vi "6229_Green_Lattice_write_waveform_2015.10.19.vi"(8 "Error In":errorcluster, 9 "Control Reference \nCluster Input":T1, 11 "6229 Green Lattice Inputs":T2={"Active Device"="6229_Green_Lattice", "Active Channels"=[TRUE, TRUE, TRUE, TRUE, FALSE, FALSE, FALSE, FALSE], "Active Phases"=[TRUE, FALSE, FALSE, FALSE, FALSE, FALSE], "Phase Times"=[1.0, 0.1, 0.1], "Trigger Channel"="/6229_Green_Lattice/PFI0", "FIFO Buffer Size"=8191.0, "Sample Step Time (us)"=0.0, "Initialization Parameters"={"Enable Initialization"=FALSE, "Initial Values"=[]}, "Waveform Parameters"=[[{"Initial Value"=1.0, "Final Value"=0.0, "Tau"=0.0, "Eta"=1.0, "Nickname"="", "Function Type"=enum."Power Law", "Conversion"=enum."B Field Grad (G/cm)", "Constant"=0.0}, {"Initial Value"=1.0, "Final Value"=0.0, "Tau"=0.0, "Eta"=1.0, "Nickname"="", "Function Type"=enum."Power Law", "Conversion"=enum."B Field Grad (G/cm)", "Constant"=0.0}, {"Initial Value"=1.0, "Final Value"=0.0, "Tau"=0.0, "Eta"=1.0, "Nickname"="", "Function Type"=enum."Power Law", "Conversion"=enum."B Field Grad (G/cm)", "Constant"=0.0}, {"Initial Value"=1.0, "Final Value"=0.0, "Tau"=0.0, "Eta"=1.0, "Nickname"="", "Function Type"=enum."Power Law", "Conversion"=enum."B Field Grad (G/cm)", "Constant"=0.0}, {"Initial Value"=1.0, "Final Value"=0.0, "Tau"=0.0, "Eta"=1.0, "Nickname"="", "Function Type"=enum."Power Law", "Conversion"=enum."B Field Grad (G/cm)", "Constant"=0.0}, {"Initial Value"=1.0, "Final Value"=0.0, "Tau"=0.0, "Eta"=1.0, "Nickname"="", "Function Type"=enum."Power Law", "Conversion"=enum."B Field Grad (G/cm)", "Constant"=0.0}], [{"Initial Value"=1.0, "Final Value"=0.0, "Tau"=0.0, "Eta"=1.0, "Nickname"="", "Function Type"=enum."Power Law", "Conversion"=enum."B Field Grad (G/cm)", "Constant"=0.0}, {"Initial Value"=1.0, "Final Value"=0.0, "Tau"=0.0, "Eta"=1.0, "Nickname"="", "Function Type"=enum."Power Law", "Conversion"=enum."B Field Grad (G/cm)", "Constant"=0.0}, {"Initial Value"=1.0, "Final Value"=0.0, "Tau"=0.0, "Eta"=1.0, "Nickname"="", "Function Type"=enum."Power Law", "Conversion"=enum."B Field Grad (G/cm)", "Constant"=0.0}, {"Initial Value"=1.0, "Final Value"=0.0, "Tau"=0.0, "Eta"=1.0, "Nickname"="", "Function Type"=enum."Power Law", "Conversion"=enum."B Field Grad (G/cm)", "Constant"=0.0}, {"Initial Value"=1.0, "Final Value"=0.0, "Tau"=0.0, "Eta"=1.0, "Nickname"="", "Function Type"=enum."Power Law", "Conversion"=enum."B Field Grad (G/cm)", "Constant"=0.0}, {"Initial Value"=1.0, "Final Value"=0.0, "Tau"=0.0, "Eta"=1.0, "Nickname"="", "Function Type"=enum."Power Law", "Conversion"=enum."B Field Grad (G/cm)", "Constant"=0.0}], [{"Initial Value"=1.0, "Final Value"=0.0, "Tau"=0.0, "Eta"=1.0, "Nickname"="", "Function Type"=enum."Power Law", "Conversion"=enum."B Field Grad (G/cm)", "Constant"=0.0}, {"Initial Value"=1.0, "Final Value"=0.0, "Tau"=0.0, "Eta"=1.0, "Nickname"="", "Function Type"=enum."Power Law", "Conversion"=enum."B Field Grad (G/cm)", "Constant"=0.0}, {"Initial Value"=1.0, "Final Value"=0.0, "Tau"=0.0, "Eta"=1.0, "Nickname"="", "Function Type"=enum."Power Law", "Conversion"=enum."B Field Grad (G/cm)", "Constant"=0.0}, {"Initial Value"=1.0, "Final Value"=0.0, "Tau"=0.0, "Eta"=1.0, "Nickname"="", "Function Type"=enum."Power Law", "Conversion"=enum."B Field Grad (G/cm)", "Constant"=0.0}, {"Initial Value"=1.0, "Final Value"=0.0, "Tau"=0.0, "Eta"=1.0, "Nickname"="", "Function Type"=enum."Power Law", "Conversion"=enum."B Field Grad (G/cm)", "Constant"=0.0}, {"Initial Value"=1.0, "Final Value"=0.0, "Tau"=0.0, "Eta"=1.0, "Nickname"="", "Function Type"=enum."Power Law", "Conversion"=enum."B Field Grad (G/cm)", "Constant"=0.0}], [{"Initial Value"=1.0, "Final Value"=0.0, "Tau"=0.0, "Eta"=1.0, "Nickname"="", "Function Type"=enum."Power Law", "Conversion"=enum."B Field Grad (G/cm)", "Constant"=0.0}, {"Initial Value"=1.0, "Final Value"=0.0, "Tau"=0.0, "Eta"=1.0, "Nickname"="", "Function Type"=enum."Power Law", "Conversion"=enum."B Field Grad (G/cm)", "Constant"=0.0}, {"Initial Value"=1.0, "Final Value"=0.0, "Tau"=0.0, "Eta"=1.0, "Nickname"="", "Function Type"=enum."Power Law", "Conversion"=enum."B Field Grad (G/cm)", "Constant"=0.0}, {"Initial Value"=1.0, "Final Value"=0.0, "Tau"=0.0, "Eta"=1.0, "Nickname"="", "Function Type"=enum."Power Law", "Conversion"=enum."B Field Grad (G/cm)", "Constant"=0.0}, {"Initial Value"=1.0, "Final Value"=0.0, "Tau"=0.0, "Eta"=1.0, "Nickname"="", "Function Type"=enum."Power Law", "Conversion"=enum."B Field Grad (G/cm)", "Constant"=0.0}, {"Initial Value"=1.0, "Final Value"=0.0, "Tau"=0.0, "Eta"=1.0, "Nickname"="", "Function Type"=enum."Power Law", "Conversion"=enum."B Field Grad (G/cm)", "Constant"=0.0}], [{"Initial Value"=1.0, "Final Value"=0.0, "Tau"=0.0, "Eta"=1.0, "Nickname"="", "Function Type"=enum."Power Law", "Conversion"=enum."B Field Grad (G/cm)", "Constant"=0.0}, {"Initial Value"=1.0, "Final Value"=0.0, "Tau"=0.0, "Eta"=1.0, "Nickname"="", "Function Type"=enum."Power Law", "Conversion"=enum."B Field Grad (G/cm)", "Constant"=0.0}, {"Initial Value"=1.0, "Final Value"=0.0, "Tau"=0.0, "Eta"=1.0, "Nickname"="", "Function Type"=enum."Power Law", "Conversion"=enum."B Field Grad (G/cm)", "Constant"=0.0}, {"Initial Value"=1.0, "Final Value"=0.0, "Tau"=0.0, "Eta"=1.0, "Nickname"="", "Function Type"=enum."Power Law", "Conversion"=enum."B Field Grad (G/cm)", "Constant"=0.0}, {"Initial Value"=1.0, "Final Value"=0.0, "Tau"=0.0, "Eta"=1.0, "Nickname"="", "Function Type"=enum."Power Law", "Conversion"=enum."B Field Grad (G/cm)", "Constant"=0.0}, {"Initial Value"=1.0, "Final Value"=0.0, "Tau"=0.0, "Eta"=1.0, "Nickname"="", "Function Type"=enum."Power Law", "Conversion"=enum."B Field Grad (G/cm)", "Constant"=0.0}], [{"Initial Value"=1.0, "Final Value"=0.0, "Tau"=0.0, "Eta"=1.0, "Nickname"="", "Function Type"=enum."Power Law", "Conversion"=enum."B Field Grad (G/cm)", "Constant"=0.0}, {"Initial Value"=1.0, "Final Value"=0.0, "Tau"=0.0, "Eta"=1.0, "Nickname"="", "Function Type"=enum."Power Law", "Conversion"=enum."B Field Grad (G/cm)", "Constant"=0.0}, {"Initial Value"=1.0, "Final Value"=0.0, "Tau"=0.0, "Eta"=1.0, "Nickname"="", "Function Type"=enum."Power Law", "Conversion"=enum."B Field Grad (G/cm)", "Constant"=0.0}, {"Initial Value"=1.0, "Final Value"=0.0, "Tau"=0.0, "Eta"=1.0, "Nickname"="", "Function Type"=enum."Power Law", "Conversion"=enum."B Field Grad (G/cm)", "Constant"=0.0}, {"Initial Value"=1.0, "Final Value"=0.0, "Tau"=0.0, "Eta"=1.0, "Nickname"="", "Function Type"=enum."Power Law", "Conversion"=enum."B Field Grad (G/cm)", "Constant"=0.0}, {"Initial Value"=1.0, "Final Value"=0.0, "Tau"=0.0, "Eta"=1.0, "Nickname"="", "Function Type"=enum."Power Law", "Conversion"=enum."B Field Grad (G/cm)", "Constant"=0.0}], [{"Initial Value"=1.0, "Final Value"=0.0, "Tau"=0.0, "Eta"=1.0, "Nickname"="", "Function Type"=enum."Power Law", "Conversion"=enum."B Field Grad (G/cm)", "Constant"=0.0}, {"Initial Value"=1.0, "Final Value"=0.0, "Tau"=0.0, "Eta"=1.0, "Nickname"="", "Function Type"=enum."Power Law", "Conversion"=enum."B Field Grad (G/cm)", "Constant"=0.0}, {"Initial Value"=1.0, "Final Value"=0.0, "Tau"=0.0, "Eta"=1.0, "Nickname"="", "Function Type"=enum."Power Law", "Conversion"=enum."B Field Grad (G/cm)", "Constant"=0.0}, {"Initial Value"=1.0, "Final Value"=0.0, "Tau"=0.0, "Eta"=1.0, "Nickname"="", "Function Type"=enum."Power Law", "Conversion"=enum."B Field Grad (G/cm)", "Constant"=0.0}, {"Initial Value"=1.0, "Final Value"=0.0, "Tau"=0.0, "Eta"=1.0, "Nickname"="", "Function Type"=enum."Power Law", "Conversion"=enum."B Field Grad (G/cm)", "Constant"=0.0}, {"Initial Value"=1.0, "Final Value"=0.0, "Tau"=0.0, "Eta"=1.0, "Nickname"="", "Function Type"=enum."Power Law", "Conversion"=enum."B Field Grad (G/cm)", "Constant"=0.0}], [{"Initial Value"=1.0, "Final Value"=0.0, "Tau"=0.0, "Eta"=1.0, "Nickname"="", "Function Type"=enum."Power Law", "Conversion"=enum."B Field Grad (G/cm)", "Constant"=0.0}, {"Initial Value"=1.0, "Final Value"=0.0, "Tau"=0.0, "Eta"=1.0, "Nickname"="", "Function Type"=enum."Power Law", "Conversion"=enum."B Field Grad (G/cm)", "Constant"=0.0}, {"Initial Value"=1.0, "Final Value"=0.0, "Tau"=0.0, "Eta"=1.0, "Nickname"="", "Function Type"=enum."Power Law", "Conversion"=enum."B Field Grad (G/cm)", "Constant"=0.0}, {"Initial Value"=1.0, "Final Value"=0.0, "Tau"=0.0, "Eta"=1.0, "Nickname"="", "Function Type"=enum."Power Law", "Conversion"=enum."B Field Grad (G/cm)", "Constant"=0.0}, {"Initial Value"=1.0, "Final Value"=0.0, "Tau"=0.0, "Eta"=1.0, "Nickname"="", "Function Type"=enum."Power Law", "Conversion"=enum."B Field Grad (G/cm)", "Constant"=0.0}, {"Initial Value"=1.0, "Final Value"=0.0, "Tau"=0.0, "Eta"=1.0, "Nickname"="", "Function Type"=enum."Power Law", "Conversion"=enum."B Field Grad (G/cm)", "Constant"=0.0}]]} {"Phase Times" format="%_3p"}) -> (0 "error out":errorcluster, 2 "counter task out":refnum<k21>, 3 "waveform task out":refnum<k21>)   [LabVIEW 2016]
uses:
  Controls/6229/6229_arb_waveform_generation.ctl
  Controls/6229/6229_evap_waveform_input.ctl
  6221 arb waveforms/6221_waveform_param.ctl
  6733_Red_MOT/Neutral_voltage_conversion_control.ctl
  6733 arb waveforms/Control 1.ctl
  <vilib>/DAQmx/write.llb/DAQmx Write (Analog 1D DBL NChan 1Samp).vi
  <vilib>/DAQmx/write.llb/DAQmx Write (Analog 1D Wfm NChan NSamp).vi
  <vilib>/DAQmx/create/channels.llb/DAQmx Create Channel (AO-Voltage-Basic).vi
  <vilib>/DAQmx/miscellaneous.llb/DAQmx Fill In Error Info.vi
  <vilib>/Waveform/WDTOps.llb/WDT Append Waveforms DBL.vi
  <vilib>/Waveform/WDTOps.llb/WDT Scale Delta t DBL.vi
  <vilib>/DAQmx/configure/timing.llb/DAQmx Timing (Sample Clock).vi
  <vilib>/DAQmx/create/channels.llb/DAQmx Create Channel (CO-Pulse Generation-Frequency).vi
  <vilib>/DAQmx/configure/timing.llb/DAQmx Timing (Implicit).vi
  <vilib>/DAQmx/configure/trigger.llb/DAQmx Start Trigger (Digital Edge).vi
  <resource>/objmgr/daqmx.rc
panel:
  out "Sample Time Delta (us)":dbl
  out "Total Time":dbl
  out "Sample Rate":dbl
  out "Waveforms":waveform(dbl)[](array[waveform])
  out "Max Sample Rate":dbl=1000000.0
  out "# Inactive Channels":i32
  out "# Active Channels":i16
  out "Inactive Channels":tag[](array[tag])
  out "Active Channels":tag[](array[tag])
  out "Samples Written":dbl
  out "Voltage Maximum":dbl
  out "Voltage Minimum":dbl
  out "AO.PhysicalChans":tag[](array[tag])
  out "Active Device":tag
  # "(0) Arm A"
  # "(1) Arm B"
  # "(2) Arm C"
  # "(3) Unused"
  # "(0) Arm A"
  # "(1) Arm B"
  # "(2) Arm C"
  # "(3) Unused"
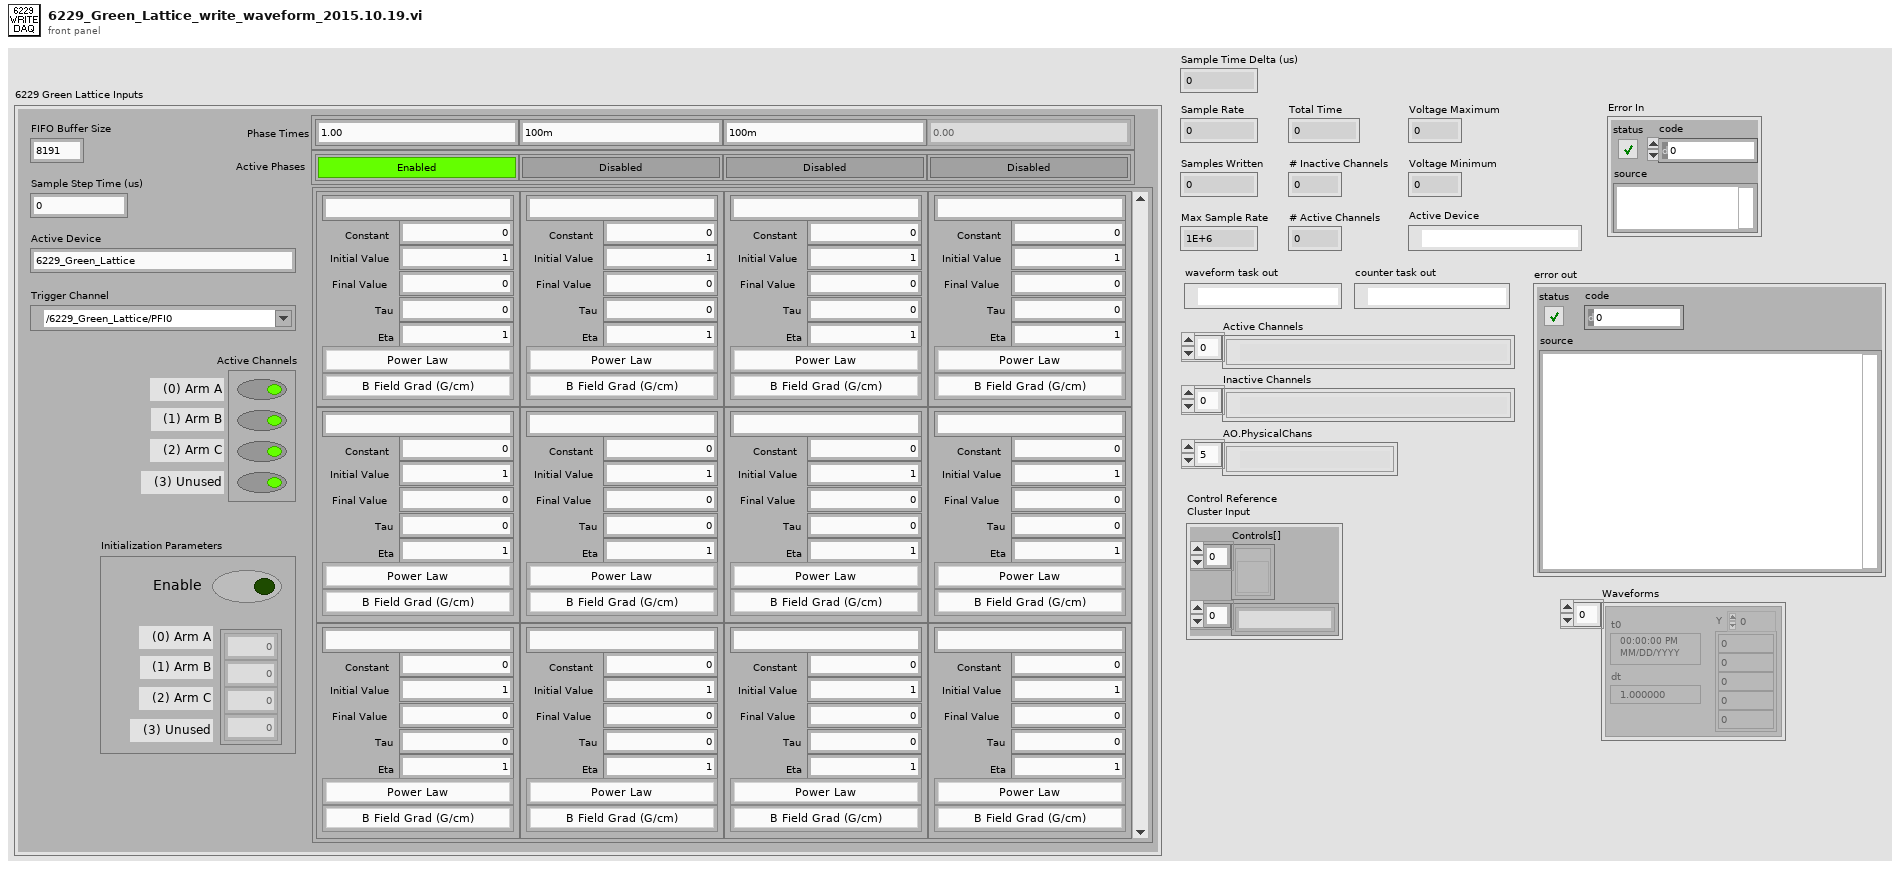
[diagram p1: front panel]
types:
  T1 = cluster{"Controls[]":refnum<vi>[], "Control Names":string[]}
  T2 = typedef "6229_arb_waveform_generation.ctl" = cluster{"Active Device":string, "Active Channels":bool[], "Active Phases":bool[], "Phase Times":dbl[], "Trigger Channel":tag, "FIFO Buffer Size":dbl, "Sample Step Time (us)":dbl, "Initialization Parameters":cluster{"Enable Initialization":bool, "Initial Values":dbl[]}, "Waveform Parameters":T3}
  T3 = typedef "6229_evap_waveform_input.ctl" = T4[][]
  T4 = typedef "6221_waveform_param.ctl" = cluster{"Initial Value":dbl, "Final Value":dbl, "Tau":dbl, "Eta":dbl, "Nickname":string, "Function Type":enum16{"Constant", "Power Law", "Evap - Calc Tau", "Evaporation Formula", "Tanh", "Exponential"}, "Conversion":T5, "Constant":dbl}
  T5 = typedef "Neutral_voltage_conversion_control.ctl" = enum16{"Volts", "B Field Grad (G/cm)", "Red Boson Cntr Freq (MHz)", "Red Boson Dither Amp (kHz)", "Red Boson Power (mW)", "Red 87 Trap Cntr Freq (MHz)", "Red 87 Trap Dither Amp (kHz)", "Red 87 Trap Power (mW)", "Red 87 Stir Cntr Freq (MHz)", "Red 87 Stir Dither Amp (kHz)", "Red 87 Stir Power (mW)", "ODT Sheet Trap Power (W)", "ODT Loading Trap Power (W)"}
  T6 = typedef "Control 1.ctl" = enum16{"Initialize", "Get Device Information", "Get Active/Inactive Channels", "Maximize Samples / Channel", "Calculate Waveforms", "Check for Problems", "Update Front Panel", "Clear Old Tasks", "Write Initialization to Cards", "Write Waveform to Cards"}
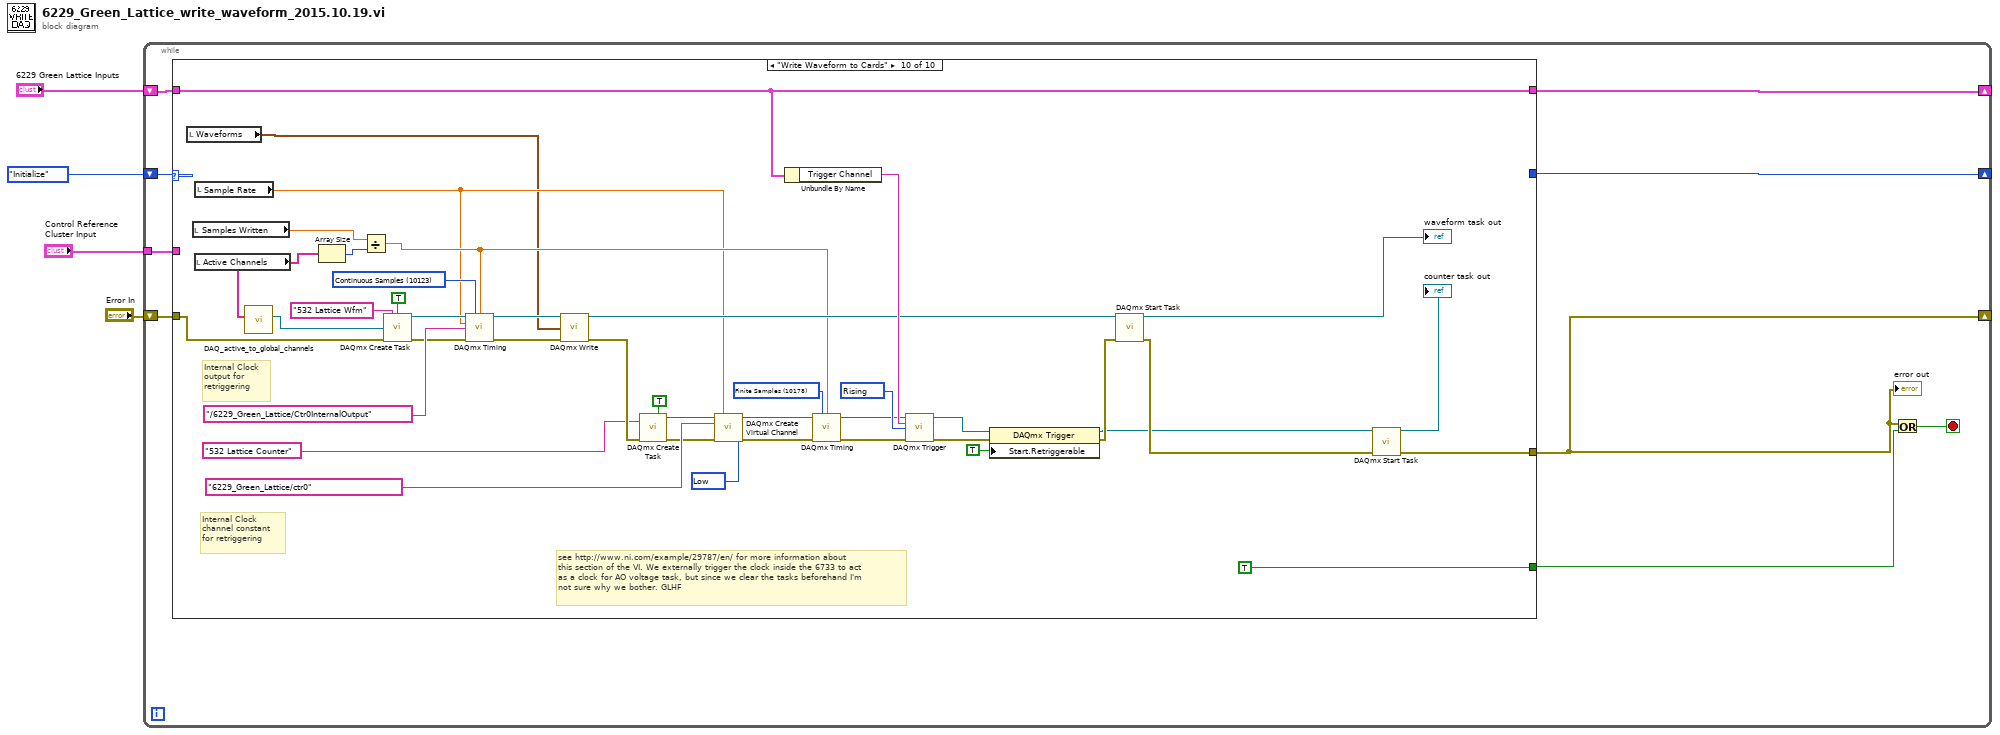
[diagram p0: block diagram]
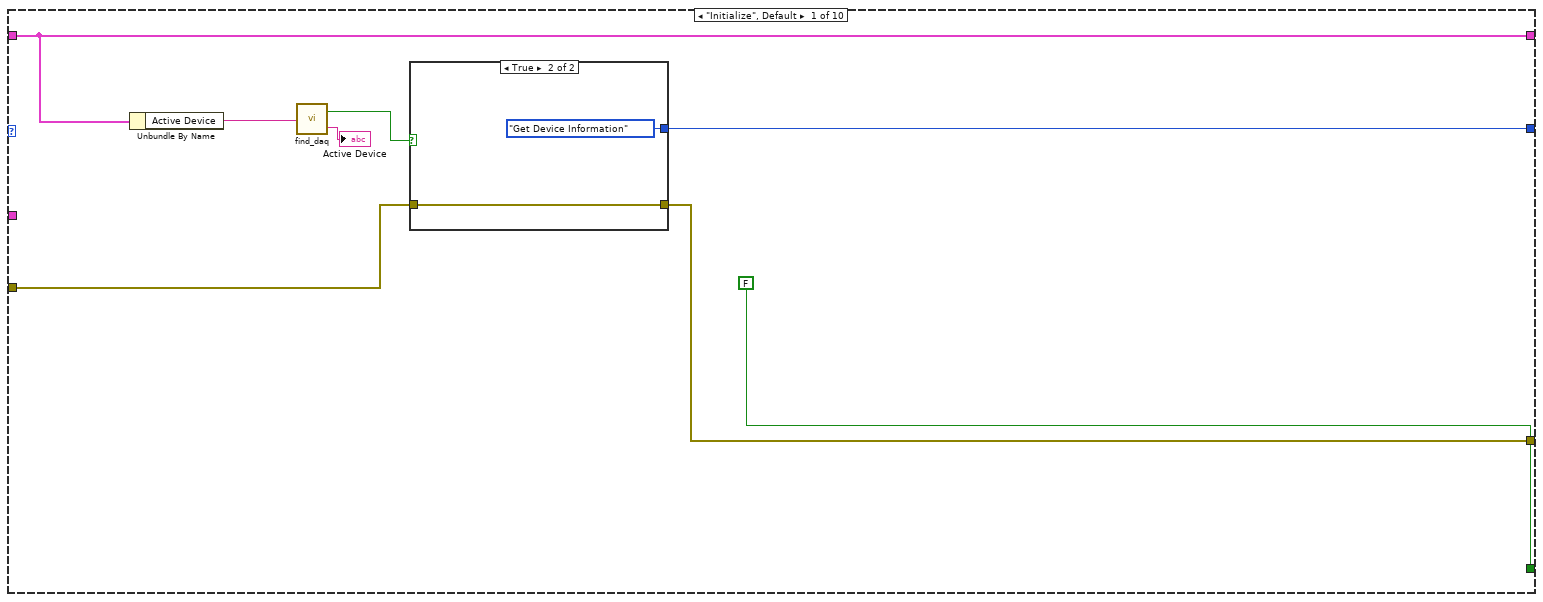
[diagram p2: hidden frame]
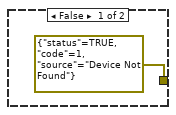
[diagram p3: hidden frame]
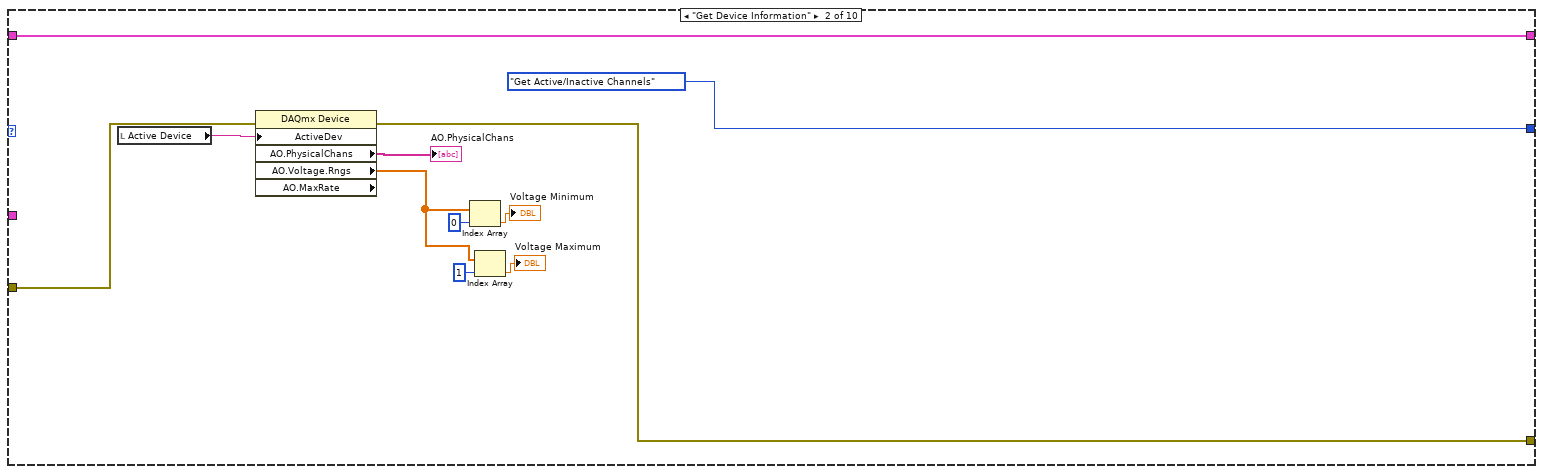
[diagram p4: hidden frame]
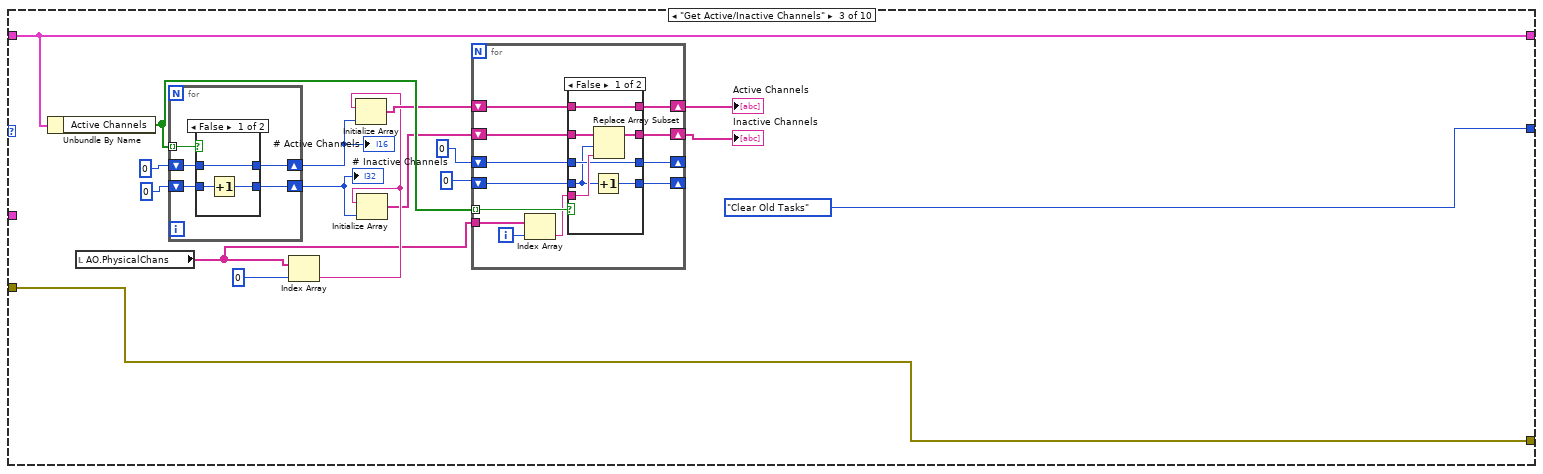
[diagram p5: hidden frame]
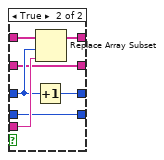
[diagram p6: hidden frame]
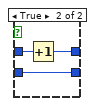
[diagram p7: hidden frame]
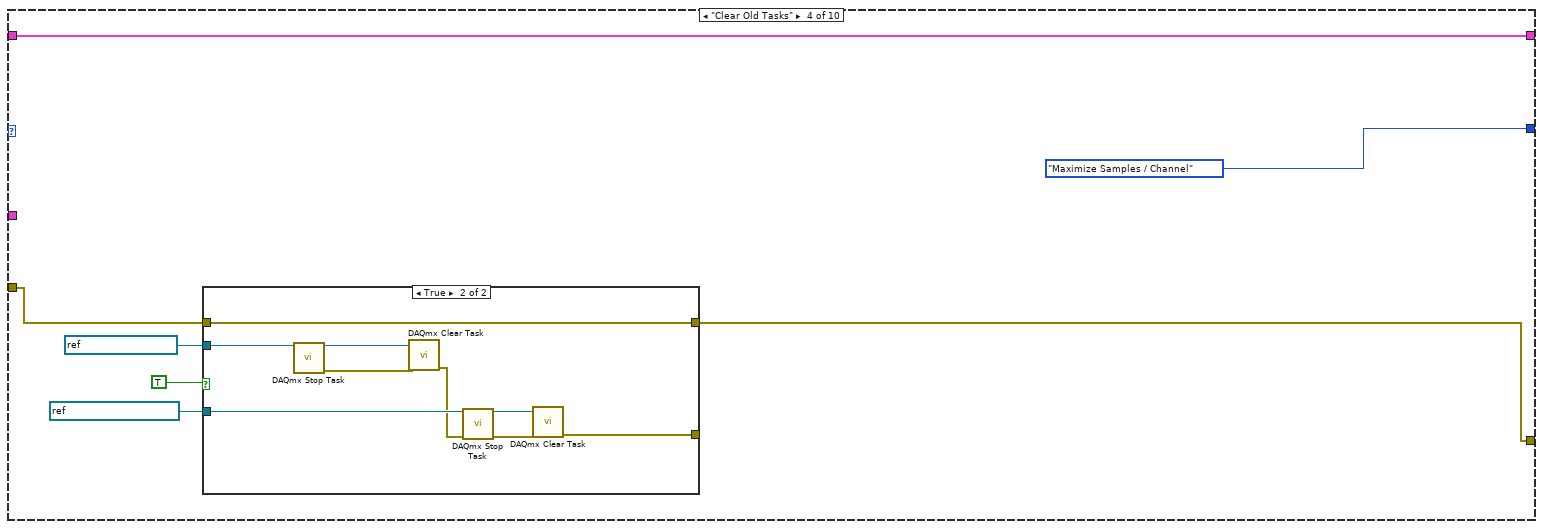
[diagram p8: hidden frame]
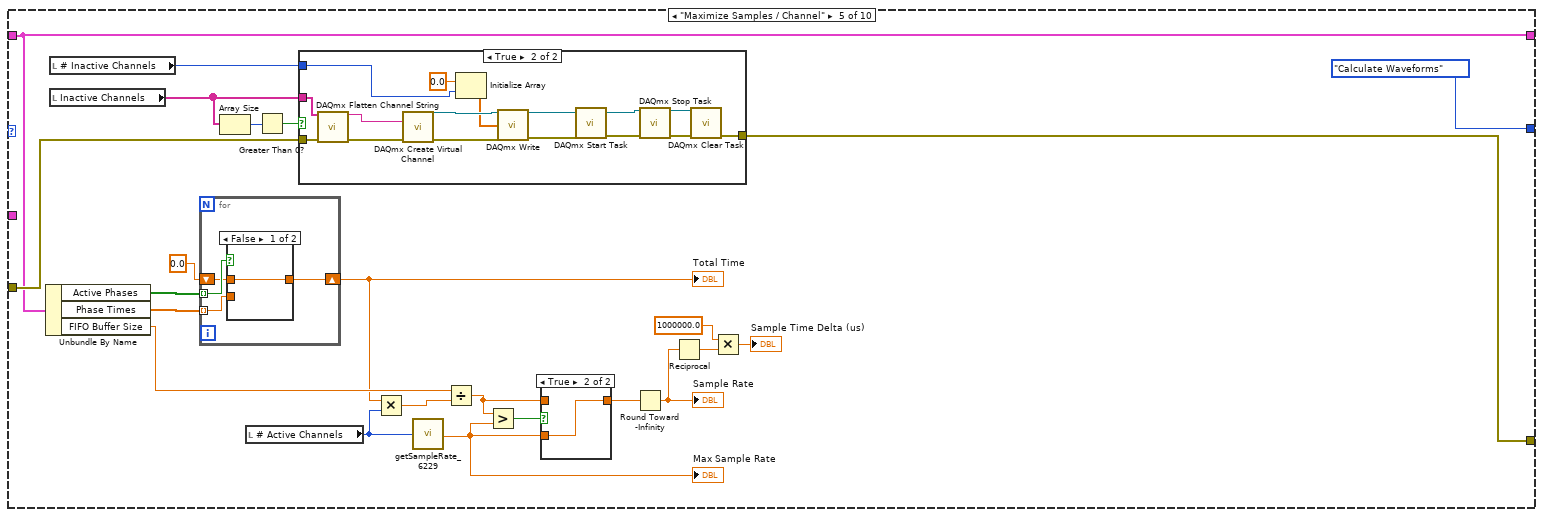
[diagram p10: hidden frame]
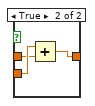
[diagram p13: hidden frame]
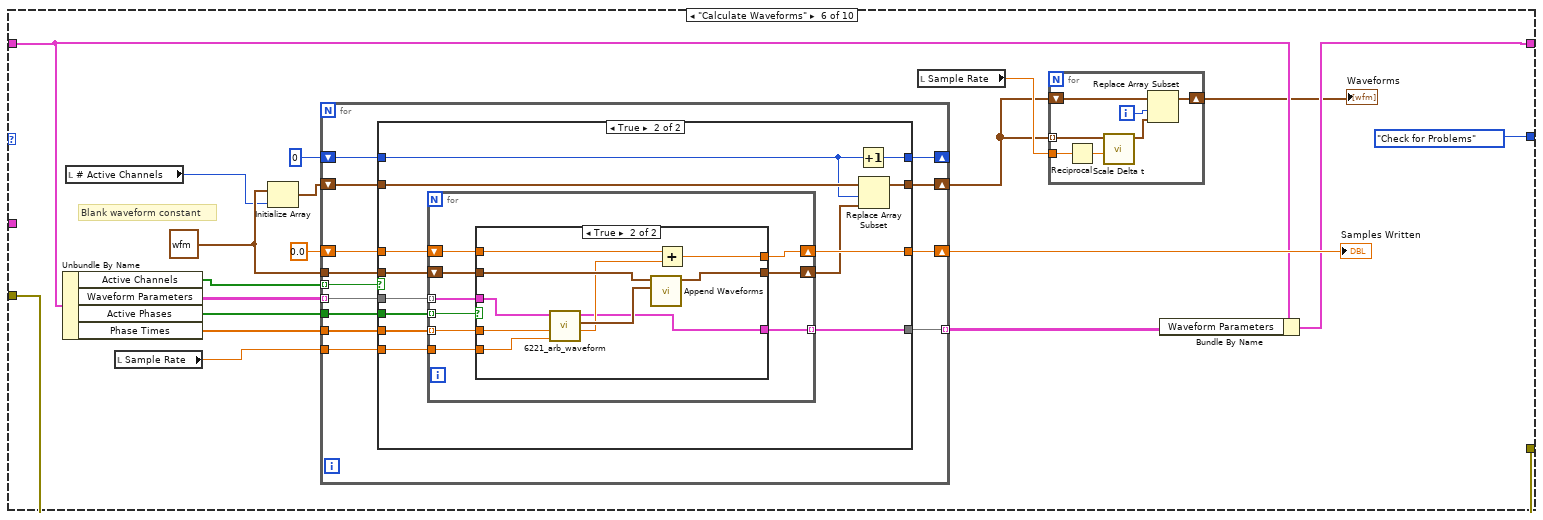
[diagram p14: hidden frame]
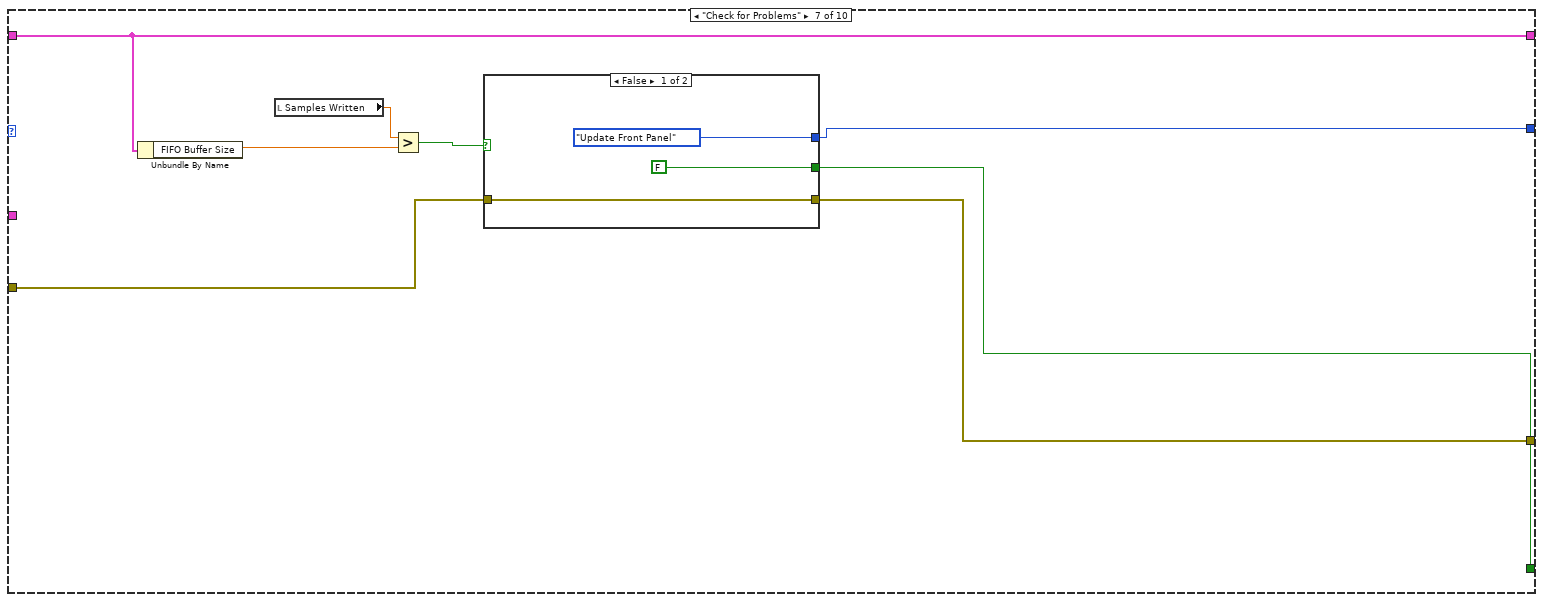
[diagram p17: hidden frame]
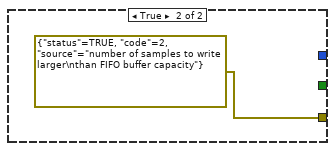
[diagram p18: hidden frame]
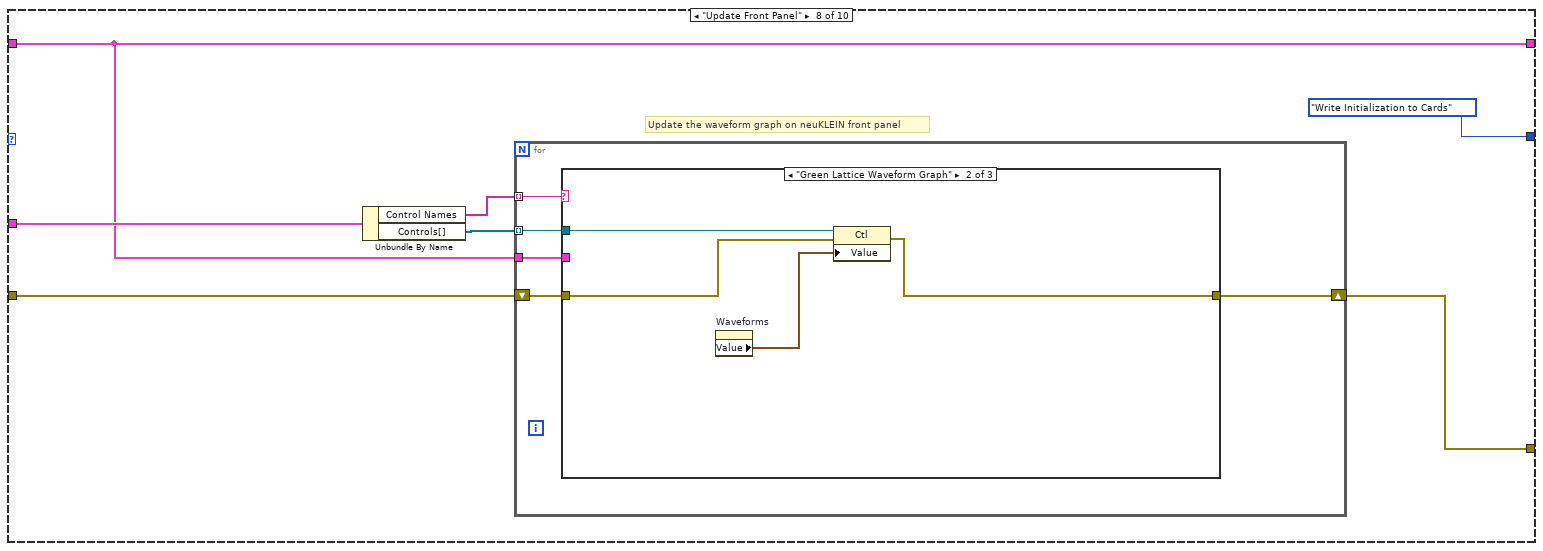
[diagram p19: hidden frame]
diagram:
  n1 = while {
    shift-right: [w9] -> _
    shift-left: "Error In" -> [w11]
    shift-right: [w10] -> _
    shift-left: Control_1."Initialize" -> [w13]
    shift-right: [w7] -> _
    shift-left: "6229 Green Lattice Inputs" -> [w12]
    tunnel: "Control Reference \nCluster Input" -> [w5]
    stop <- w8 stop-if-true
    n2 = case shown="\"Write Waveform to Cards\"" w13 {
      tunnel: w12 -> [w15 w35 w39 w92 w114 w163 w235 w248 w281 w345]
      tunnel: [w18 w27 w50 w95 w127 w174 w240 w249 w283 w326] -> w9
      tunnel: w11 -> [w17 w34 w50 w94 w129 w174 w241 w250 w285 w323]
      tunnel: [w16 Control_1."Get Active/Inactive Channels" Control_1."Clear Old Tasks" Control_1."Maximize Samples / Channel" Control_1."Calculate Waveforms" Control_1."Check for Problems" w239 Control_1."Write Initialization to Cards" Control_1."Write Waveform to Cards" _] -> w10
      tunnel: [w15 w35 w39 w92 w114 w162 w235 w248 w281 w345] -> w7
      tunnel: [FALSE ("y") _ _ _ _ _ w238 _ _ TRUE ("y")] -> w6
      tunnel: w5 -> [_ _ _ _ _ _ _ w251 _ _]
      frame "Initialize", Default {
        n3 = Unbundle By Name(w15) -> ("Active Device"=w21:string)
        n4 = call "find_daq.vi"("Device Name"=w21) -> ("Device Present"=w19:bool, "DAQmx Device Name"=→"Active Device":tag)
        n5 = case shown="True" w19 {
          tunnel: [errorcluster {"status"=TRUE, "code"=1, "source"="Device Not Found"} ("error in (no error)") w24] -> w18
          tunnel: w17 -> [_ w24]
          tunnel: [_ Control_1."Get Device Information"] -> w16
          frame False {
          }
          frame True {
          }
        }
      }
      frame "Get Device Information" {
        n6 = local read "Active Device"() -> (w25:tag)
        n7 = property class="DAQmx Device" props=["ActiveDev", "AO.PhysicalChans", "AO.Voltage.Rngs", "AO.MaxRate"](error in=w34, "ActiveDev"=w25) -> (error out=w27:errorcluster, "AO.PhysicalChans"=→"AO.PhysicalChans":tag[], "AO.Voltage.Rngs"=w29:dbl[])  [unwired: 1 in, 2 out]
        n8 = Index Array(array=w29, index=0) -> (element=→"Voltage Minimum":dbl)
        n9 = Index Array(array=w29, index=1) -> (element=→"Voltage Maximum":dbl)
      }
      frame "Get Active/Inactive Channels" {
        n10 = Unbundle By Name(w39) -> ("Active Channels"=w49:bool[])
        n11 = local read "AO.PhysicalChans"() -> (w43:tag[])
        n12 = for {
          shift-right: [w83] -> w48
          shift-left: i16 0 -> [w82]
          shift-right: [w81] -> w47
          shift-left: 0 -> [w80]
          tunnel: w49 -> [w79] mode=indexing
          n13 = case shown="False" w79 {
            tunnel: [w84 w89] -> w83
            tunnel: w82 -> [w84 w88]
            tunnel: [w86 w87] -> w81
            tunnel: w80 -> [w85 w87]
            frame False {
              n14 = Increment(x=w85) -> (x+1=w86:i32)
            }
            frame True {
              n15 = Increment(x=w88) -> (x+1=w89:i16)
            }
          }
        }
        "# Active Channels" <- w48
        "# Inactive Channels" <- w47
        n16 = Index Array(array=w43, index=0) -> (element=w44:tag)
        n17 = Initialize Array(w44, w48) -> (w46:tag[])
        n18 = Initialize Array(w44, w47) -> (w42:tag[])
        n19 = for {
          tunnel: w49 -> [w64] mode=indexing
          shift-right: [w61] -> w38
          shift-left: w46 -> [w62]
          tunnel: w43 -> [w59]
          shift-right: [w57] -> w37
          shift-left: w42 -> [w58]
          shift-right: [w55] -> _
          shift-left: 0 ("index") -> [w56]
          shift-right: [w53] -> _
          shift-left: 0 ("index") -> [w54]
          i -> [w63]
          n20 = Index Array(array=w59, index=w63) -> (element=w60:tag)
          n21 = case shown="False" w64 {
            tunnel: w62 -> [w65 w78]
            tunnel: [w65 w77] -> w61
            tunnel: w60 -> [w71 w76]
            tunnel: w58 -> [w70 w72]
            tunnel: [w69 w72] -> w57
            tunnel: w56 -> [w68 w75]
            tunnel: [w68 w74] -> w55
            tunnel: w54 -> [w67 w73]
            tunnel: [w66 w73] -> w53
            frame False {
              n22 = Increment(x=w67) -> (x+1=w66:i32)
              n23 = Replace Array Subset(array=w70, new element=w71, index=w67) -> (w69:tag[])
            }
            frame True {
              n24 = Increment(x=w75) -> (x+1=w74:i32)
              n25 = Replace Array Subset(array=w78, new element=w76, index=w75) -> (w77:tag[])
            }
          }
        }
        "Active Channels" <- w38
        "Inactive Channels" <- w37
      }
      frame "Clear Old Tasks" {
        n26 = case shown="True" TRUE {
          tunnel: refnum<k21> "532 Lattice Wfm" ("Waveform Task In") -> [_ w106]
          tunnel: refnum<k21> "532 Lattice Counter" ("Control Task In") -> [_ w104]
          tunnel: [w97 w102] -> w95
          tunnel: w94 -> [w97 w102]
          tunnel: [_ w98] -> _
          frame False {
          }
          frame True {
            n27 = call <vilib>:"DAQmx Stop Task.vi"("task/channels in"=w106) -> ("task out"=w105:refnum<k21>, "error out"=w101:errorcluster)  [unwired: 13 in]
            n28 = call <vilib>:"DAQmx Clear Task.vi"("task in"=w105, "error in"=w101) -> ("error out"=w100:errorcluster)  [unwired: 13 in]
            n29 = call <vilib>:"DAQmx Stop Task.vi"("task/channels in"=w104, "error in"=w100) -> ("task out"=w103:refnum<k21>, "error out"=w99:errorcluster)  [unwired: 12 in]
            n30 = call <vilib>:"DAQmx Clear Task.vi"("task in"=w103, "error in"=w99) -> ("error out"=w98:errorcluster)  [unwired: 13 in]
          }
        }
      }
      frame "Maximize Samples / Channel" {
        n31 = Unbundle By Name(w114) -> ("Active Phases"=w125:bool[], "Phase Times"=w124:dbl[], "FIFO Buffer Size"=w117:dbl)
        n32 = local read "# Inactive Channels"() -> (w128:i32)
        n33 = local read "Inactive Channels"() -> (w113:tag[])
        n34 = for {
          tunnel: w125 -> [w152] mode=indexing
          tunnel: w124 -> [w151] mode=indexing
          shift-right: [w149] -> w116
          shift-left: 0.0 -> [w150]
          n35 = case shown="False" w152 {
            tunnel: w151 -> [_ w156]
            tunnel: w150 -> [w153 w155]
            tunnel: [w153 w154] -> w149
            frame False {
            }
            frame True {
              n36 = Add(x=w156, y=w155) -> (x+y=w154:dbl)
            }
          }
        }
        "Total Time" <- w116
        n37 = Array Size(array=w113) -> (size(s)=w112:i32)
        n38 = local read "# Active Channels"() -> (w115:i16)
        n39 = Greater Than 0?(x=w112) -> (x > 0?=w111:bool)
        n40 = case shown="True" w111 {
          tunnel: w129 -> [w130 w145]
          tunnel: w128 -> [_ w139]
          tunnel: [w130 w134] -> w127
          tunnel: w113 -> [_ w131]
          frame False {
          }
          frame True {
            n41 = call <vilib>:"DAQmx Flatten Channel String.vi"("names in"=w131, "error in"=w145) -> ("names out"=w144:string, "error out"=w146:errorcluster)  [unwired: 12 in]
            n42 = call-poly <vilib>:"DAQmx Create Virtual Channel.vi"("physical channels"=w144, "error in"=w146) -> ("task out"=w143:refnum<k21>, "error out"=w142:errorcluster)  [unwired: 12 in]
            n43 = Initialize Array(0.0 ("element"), w139) -> (w137:dbl[])
            n44 = call-poly <vilib>:"DAQmx Write.vi"("task/channels in"=w143, "data"=w137, "error in"=w142) -> ("task out"=w140:refnum<k21>, "error out"=w141:errorcluster)  [unwired: 10 in, 1 out]
            n45 = call <vilib>:"DAQmx Start Task.vi"("task/channels in"=w140, "error in"=w141) -> ("task out"=w132:refnum<k21>, "error out"=w133:errorcluster)  [unwired: 12 in]
            n46 = call <vilib>:"DAQmx Stop Task.vi"("task/channels in"=w132, "error in"=w133) -> ("task out"=w136:refnum<k21>, "error out"=w135:errorcluster)  [unwired: 12 in]
            n47 = call <vilib>:"DAQmx Clear Task.vi"("task in"=w136, "error in"=w135) -> ("error out"=w134:errorcluster)  [unwired: 13 in]
          }
        }
        n48 = Multiply(x=w116, y=w115) -> (x*y=w121:dbl)
        n49 = call "getSampleRate_6229.vi"("Number of active channels"=w115) -> ("Sample Rate"=w120:dbl)
        "Max Sample Rate" <- w120
        n50 = Divide(x=w117, y=w121) -> (x/y=w119:dbl)
        n51 = Greater?(x=w119, y=w120) -> (0:w122:bool)
        n52 = case shown="True" w122 {
          tunnel: [w147 w148] -> w118
          tunnel: w120 -> [_ w148]
          tunnel: w119 -> [w147 _]
          frame False {
          }
          frame True {
          }
        }
        n53 = Round Toward -Infinity(1:w118) -> (0:w110:dbl)
        "Sample Rate" <- w110
        n54 = Reciprocal(x=w110) -> (1/x=w109:dbl)
        n55 = Multiply(x=1000000.0, y=w109) -> (x*y=→"Sample Time Delta (us)":dbl)
      }
      frame "Calculate Waveforms" {
        w169 = waveform(dbl) {"t0"=timestamp(0 s since 1904-01-01), "dt"=1.0, "Y"=[]}
        # "Blank waveform constant"
        n56 = Unbundle By Name(w163) -> ("Active Channels"=w166:bool[], "Waveform Parameters"=w175:T3, "Active Phases"=w170:bool[], "Phase Times"=w167:dbl[])
        n57 = local read "# Active Channels"() -> (w164:i16)
        n58 = local read "Sample Rate"() -> (w165:dbl)
        n59 = Initialize Array(w169, w164) -> (w168:waveform(dbl)[])
        n60 = for {
          tunnel: w166 -> [w195] mode=indexing
          tunnel: w175 -> [w194] mode=indexing
          shift-right: [w193] -> w173
          shift-left: 0.0 -> [w192]
          tunnel: w170 -> [w191]
          tunnel: w169 -> [w190]
          shift-right: [w188] -> w158
          shift-left: w168 -> [w189]
          tunnel: w167 -> [w187]
          tunnel: w165 -> [w186]
          tunnel: [w185] -> w161 mode=indexing
          shift-right: [w183] -> _
          shift-left: 0 -> [w184]
          n61 = case shown="True" w195 {
            tunnel: w184 -> [w196 w201]
            tunnel: w194 -> [w197 w202]
            tunnel: [w199 w212] -> w193
            tunnel: w192 -> [w199 w211]
            tunnel: w191 -> [_ w210]
            tunnel: w190 -> [_ w209]
            tunnel: w189 -> [w198 w208]
            tunnel: [w198 w207] -> w188
            tunnel: w187 -> [_ w206]
            tunnel: w186 -> [_ w205]
            tunnel: [w197 w203] -> w185
            tunnel: [w196 w200] -> w183
            frame False {
            }
            frame True {
              n62 = for {
                shift-right: [w221] -> w212
                shift-left: w211 -> [w220]
                tunnel: w202 -> [w219] mode=indexing
                shift-right: [w217] -> w204
                shift-left: w209 -> [w218]
                tunnel: w210 -> [w216] mode=indexing
                tunnel: w206 -> [w215] mode=indexing
                tunnel: w205 -> [w214]
                tunnel: [w213] -> w203 mode=indexing
                n63 = case shown="True" w216 {
                  tunnel: [w224 w234] -> w221
                  tunnel: w220 -> [w224 w233]
                  tunnel: w219 -> [w222 w228]
                  tunnel: w218 -> [w223 w232]
                  tunnel: [w223 w231] -> w217
                  tunnel: w215 -> [_ w229]
                  tunnel: w214 -> [_ w230]
                  tunnel: [w222 w225] -> w213
                  frame False {
                  }
                  frame True {
                    n64 = call "6221_arb_waveform.vi"("Waveform Input"=w228, "Phase Time"=w229, "Sample Rate"=w230) -> ("Waveform Output"=w225:T4, "output waveform"=w227:waveform(dbl), "# Samples"=w226:dbl)  [unwired: 5 in]
                    n65 = call-poly <vilib>:"Append Waveforms.vi"("waveform B"=w227, "waveform A"=w232) -> ("waveform out"=w231:waveform(dbl))  [unwired: 8 in, 1 out]
                    n66 = Add(x=w233, y=w226) -> (x+y=w234:dbl)
                  }
                }
              }
              n67 = Increment(x=w201) -> (x+1=w200:i32)
              n68 = Replace Array Subset(array=w208, new element=w204, index=w201) -> (w207:waveform(dbl)[])
            }
          }
        }
        "Samples Written" <- w173
        n69 = local read "Sample Rate"() -> (w159:dbl)
        n70 = for {
          shift-right: [w179] -> w157
          shift-left: w158 -> [w177]
          tunnel: w159 -> [w178]
          tunnel: w158 -> [w176] mode=indexing
          i -> [w181]
          n71 = Reciprocal(x=w178) -> (1/x=w182:dbl)
          n72 = call-poly <vilib>:"Scale Delta t.vi"("scale factor"=w182, "waveform in"=w176) -> ("waveform out"=w180:waveform(dbl))  [unwired: 8 in, 1 out]
          n73 = Replace Array Subset(array=w177, new element=w180, index=w181) -> (w179:waveform(dbl)[])
        }
        "Waveforms" <- w157
        n74 = Bundle By Name(cluster=w163, "Waveform Parameters"=w161) -> (w162:T2)
      }
      frame "Check for Problems" {
        n75 = Unbundle By Name(w235) -> ("FIFO Buffer Size"=w236:dbl)
        n76 = local read "Samples Written"() -> (w237:dbl)
        n77 = Greater?(x=w237, y=w236) -> (0:w242:bool)
        n78 = case shown="False" w242 {
          tunnel: w241 -> [w245 _]
          tunnel: [w245 errorcluster {"status"=TRUE, "code"=2, "source"="number of samples to write larger\nthan FIFO buffer capacity"} ("error in (no error)")] -> w240
          tunnel: [Control_1."Update Front Panel" _] -> w239
          tunnel: [FALSE ("y") _] -> w238
          frame False {
          }
          frame True {
          }
        }
      }
      frame "Update Front Panel" {
        # "Update the waveform graph on neuKLEIN front panel"
        n79 = Unbundle By Name(w251) -> ("Control Names"=w253:string[], "Controls[]"=w252:refnum<vi>[])
        n80 = for {
          tunnel: w253 -> [w258] mode=indexing
          shift-right: [w255] -> w249
          shift-left: w250 -> [w256]
          tunnel: w252 -> [w257] mode=indexing
          tunnel: w248 -> [w254]
          n81 = case shown="\"Green Lattice Waveform Graph\"" w258 {
            tunnel: w257 -> [_ w261 w269]
            tunnel: w256 -> [w259 w263 w271]
            tunnel: [w259 w262 w270] -> w255
            tunnel: w254 -> [_ _ w268]
            frame "False", Default {
            }
            frame "Green Lattice Waveform Graph" {
              n82 = property on="Waveforms" class="Arr (strict)"() -> ("Value"=w260:waveform(dbl)[])  [unwired: 2 in, 2 out]
              n83 = property class="Ctl"(reference=w261, error in=w263, "Value"=w260) -> (error out=w262:errorcluster)  [unwired: 1 out]
            }
            frame "6229 Green Lattice Inputs" {
              n84 = local read "Sample Rate"() -> (w264:dbl)
              n85 = Unbundle By Name(w268) -> ("Waveform Parameters"=w272:T3)
              n86 = Reciprocal(x=w264) -> (1/x=w267:dbl)
              n87 = Multiply(x=1000000.0, y=w267) -> (x*y=w265:dbl)
              n88 = property class="Ctl"(reference=w269, error in=w271) -> (reference out=w276:refnum<vi>, error out=w274:errorcluster, "Value"=w278:variant)
              n89 = Variant To Data(error in=w274, type=w268, Variant=w278) -> (data=w277:T2, error out=w273:errorcluster)
              n90 = Bundle By Name(cluster=w277, "Waveform Parameters"=w272, "Sample Step Time (us)"=w265) -> (w275:T2)
              n91 = property class="Ctl"(reference=w276, error in=w273, "Value"=w275) -> (error out=w270:errorcluster)  [unwired: 1 out]
            }
          }
        }
      }
      frame "Write Initialization to Cards" {
        n92 = Unbundle By Name(w281) -> ("Initialization Parameters.Enable Initialization"=w282:bool, "Initialization Parameters.Initial Values"=w280:dbl[], "Active Channels"=w279:bool[])
        n93 = case shown="True" w282 {
          tunnel: w285 -> [w286 w301]
          tunnel: [w286 w291] -> w283
          tunnel: w280 -> [_ w288]
          tunnel: w279 -> [_ w289]
          frame False {
          }
          frame True {
            n94 = for {
              tunnel: w288 -> [w304] mode=indexing
              tunnel: w289 -> [w303] mode=indexing
              tunnel: [w304] -> w287 mode=indexing if=w303
            }
            n95 = local read "Active Channels"() -> (w302:tag[])
            n96 = call "DAQ_active_to_global_channels.vi"("Active Channels"=w302) -> ("Global Channels"=w300:refnum<k21>)  [unwired: 10 in]
            n97 = call <vilib>:"DAQmx Create Task.vi"("new task name"="532 Lattice Init", "auto cleanup"=FALSE, "global virtual channels"=w300, "error in"=w301) -> ("task out"=w299:refnum<k21>, "error out"=w298:errorcluster)  [unwired: 10 in]
            n98 = call-poly <vilib>:"DAQmx Write.vi"("task/channels in"=w299, "auto start"=TRUE, "data"=w287, "error in"=w298) -> ("task out"=w290:refnum<k21>, "error out"=w292:errorcluster)  [unwired: 9 in, 1 out]
            n99 = call <vilib>:"DAQmx Stop Task.vi"("task/channels in"=w290, "error in"=w292) -> ("task out"=w294:refnum<k21>, "error out"=w293:errorcluster)  [unwired: 12 in]
            n100 = call <vilib>:"DAQmx Clear Task.vi"("task in"=w294, "error in"=w293) -> ("error out"=w291:errorcluster)  [unwired: 13 in]
          }
        }
      }
      frame "Write Waveform to Cards" {
        w311 = 10178 items=["Finite Samples"=10178, "Continuous Samples"=10123, "Hardware Timed Single Point"=12522] ("sample mode")
        w337 = 10280 items=["Rising"=10280, "Falling"=10171] ("edge")
        w341 = 10123 items=["Finite Samples"=10178, "Continuous Samples"=10123, "Hardware Timed Single Point"=12522] ("sample mode")
        w344 = 10214 items=["High"=10192, "Low"=10214] ("idle state")
        # "see http://www.ni.com/example/29787/en/ for more information about\nthis section of the VI. We externally trigger the clock inside the 6733 to act\nas a clock for AO voltage task, but since we clear the tasks beforehand I'm\nnot sure why we bother. GLHF"
        # "Internal Clock\noutput for\nretriggering"
        # "Internal Clock\nchannel constant\nfor retriggering"
        n101 = local read "Waveforms"() -> (w305:waveform(dbl)[])
        n102 = local read "Samples Written"() -> (w309:dbl)
        n103 = local read "Active Channels"() -> (w308:tag[])
        n104 = local read "Sample Rate"() -> (w306:dbl)
        n105 = call "DAQ_active_to_global_channels.vi"("Active Channels"=w308) -> ("Global Channels"=w321:refnum<k21>)  [unwired: 10 in]
        n106 = Array Size(array=w308) -> (size(s)=w310:i32)
        n107 = Divide(x=w309, y=w310) -> (x/y=w307:dbl)
        n108 = call <vilib>:"DAQmx Create Task.vi"("new task name"="532 Lattice Wfm", "auto cleanup"=TRUE, "global virtual channels"=w321, "error in"=w323) -> ("task out"=w319:refnum<k21>, "error out"=w322:errorcluster)  [unwired: 10 in]
        n109 = call-poly <vilib>:"DAQmx Timing.vi"("task/channels in"=w319, "sample mode"=w341, "samples per channel"=w307, "rate"=w306, "source"=tag "/6229_Green_Lattice/Ctr0InternalOutput", "error in"=w322) -> ("task out"=w339:refnum<k21>, "error out"=w340:errorcluster)  [unwired: 8 in]
        n110 = call-poly <vilib>:"DAQmx Write.vi"("task/channels in"=w339, "data"=w305, "error in"=w340) -> ("task out"=w331:refnum<k21>, "error out"=w318:errorcluster)  [unwired: 10 in, 1 out]
        n111 = call <vilib>:"DAQmx Create Task.vi"("new task name"="532 Lattice Counter", "auto cleanup"=TRUE, "error in"=w318) -> ("task out"=w313:refnum<k21>, "error out"=w317:errorcluster)  [unwired: 11 in]
        n112 = call-poly <vilib>:"DAQmx Create Virtual Channel.vi"("task in"=w313, "frequency"=w306, "counter"=tag "6229_Green_Lattice/ctr0", "error in"=w317, "idle state"=w344) -> ("task out"=w343:refnum<k21>, "error out"=w342:errorcluster)  [unwired: 9 in]
        n113 = Unbundle By Name(w345) -> ("Trigger Channel"=w336:tag)
        n114 = call-poly <vilib>:"DAQmx Timing.vi"("task/channels in"=w343, "sample mode"=w311, "samples per channel"=w307, "error in"=w342) -> ("task out"=w335:refnum<k21>, "error out"=w338:errorcluster)  [unwired: 10 in]
        n115 = call-poly <vilib>:"DAQmx Trigger.vi"("task/channels in"=w335, "source"=w336, "edge"=w337, "error in"=w338) -> ("task out"=w333:refnum<k21>, "error out"=w334:errorcluster)  [unwired: 10 in]
        n116 = property class="DAQmx Trigger"(reference=w333, error in=w334, "Start.Retriggerable"=TRUE) -> (reference out=w312:refnum<k21>, error out=w330:errorcluster)
        n117 = call <vilib>:"DAQmx Start Task.vi"("task/channels in"=w331, "error in"=w330) -> ("task out"=→"waveform task out":refnum<k21>, "error out"=w329:errorcluster)  [unwired: 12 in]
        n118 = call <vilib>:"DAQmx Start Task.vi"("task/channels in"=w312, "error in"=w329) -> ("task out"=→"counter task out":refnum<k21>, "error out"=w326:errorcluster)  [unwired: 12 in]
      }
    }
    "error out" <- w9
    n119 = Or(x=w9, y=w6) -> (x .or. y?=w8:bool)
  }
